vi "双while.vi"() -> ()   [LabVIEW 2018]
panel:
  in  "数值":dbl
  in  "停止":bool
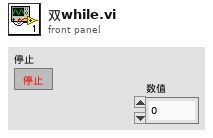
[diagram p1: front panel]
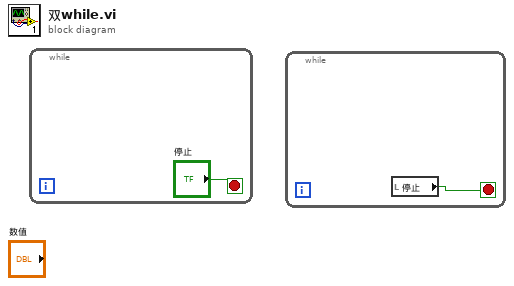
[diagram p0: block diagram]
diagram:
  n1 = while {
    stop <- "停止" stop-if-true
  }
  n2 = while {
    stop <- w2 stop-if-true
    n3 = local read "停止"() -> (w2:bool)
  }
